vi "Write Key.vi"   [LabVIEW 2020, in "NI_LVConfig.lvlib"]
doc: "Writes a value to a key in a specified section of the configuration data identified by <B>refnum</B>. This VI modifies data in memory. To write data to disk, use the Close Config Data VI. Wire data to the <B>value</B> input to determine the polymorphic instance to use or manually select the instance."
uses:
  <vilib>/Utility/config.llb/NI_LVConfig.lvlib
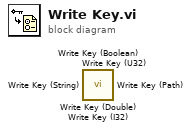
[diagram p0: block diagram]
diagram:
  n1 = call "Write Key (Double).vi"() -> ()  [unwired: 9 in, 3 out]
  n2 = call <vilib>:"Write Key (U32).vi"() -> ()  [unwired: 9 in, 3 out]
  n3 = call <vilib>:"Write Key (String).vi"() -> ()  [unwired: 9 in, 3 out]
  n4 = call <vilib>:"Write Key (Path).vi"() -> ()  [unwired: 9 in, 3 out]
  n5 = call <vilib>:"Write Key (I32).vi"() -> ()  [unwired: 9 in, 3 out]
  n6 = call <vilib>:"Write Key (Boolean).vi"() -> ()  [unwired: 9 in, 3 out]
